vi "niFPGA Boolean Crossing.vi"(2 "input":bool, 3 "direction":enum8{"either", "false-true", "true-false"}(ring), 5 "initialize":bool) -> (7 "crossing":bool)   [LabVIEW 2017]
doc: "Detects state changes of Boolean input points. You can choose from three detectors: either, false-true, or true-false."
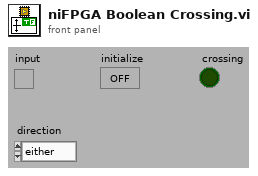
[diagram p1: front panel]
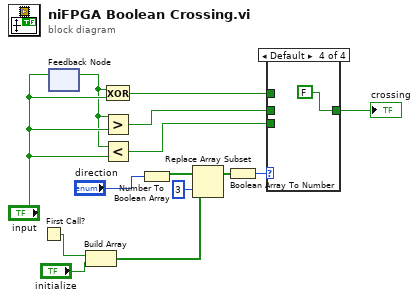
[diagram p0: block diagram]
diagram:
  n1 = First Call?() -> (First Call?: T/F=w2:bool)
  n2 = feedback-in #1("input") -> ()
  n3 = feedback #1() -> (w12:bool)  [unwired: 1 in]
  n4 = Build Array(w2, "initialize") -> (w6:bool[])
  n5 = Exclusive Or(1:"input", 2:w12) -> (0:w11:bool)
  n6 = Greater?(x=w12, y="input") -> (0:w10:bool)
  n7 = Less?(x=w12, y="input") -> (x < y?=w9:bool)
  n8 = Number To Boolean Array(number="direction") -> (Boolean array=w8:bool[])
  n9 = Replace Array Subset(array=w8, new element=w6, index=u8 3) -> (w4:bool[])
  n10 = Boolean Array To Number(Boolean array=w4) -> (number=w5:u8)
  n11 = case shown="Default" w5 {
    tunnel: [w15 w16 w17 FALSE] -> w1
    tunnel: w11 -> [w15 _ _ _]
    tunnel: w10 -> [_ w16 _ _]
    tunnel: w9 -> [_ _ w17 _]
    frame 0 {
    }
    frame 2 {
    }
    frame 1 {
    }
    frame Default {
    }
  }
  "crossing" <- w1
